vi "KE622x -- Set Lin Log Sweep Params.vi"(0 "Resource In":refnum<visa-resource-name>, 1 "Check For SCPI Errors? (T)":bool=TRUE, 7 "Lin Log Sweep Params In":T1={"Sweep Type"=enum."Linear", "Source Delay (s)"=0.001, "Range Method"=enum."Fixed", "Num Sweeps"=enum."Sweep Count", "Sweep Count"=1, "Start Level (A)"=0.0, "Stop Level (A)"=0.1, "Step Level (A)"=0.01, "Num Steps"=11, "Abort On\nCompliance?"=FALSE} {"Num Steps" min=1 max=65535; "Step Level (A)" min=-0.105 max=0.105 format="%.4p"; "Stop Level (A)" min=-0.105 max=0.105 format="%.4p"; "Start Level (A)" min=-0.105 max=0.105 format="%.4p"; "Sweep Count" min=1 max=9999; "Source Delay (s)" min=0.001 max=1000.0 step=0.001 format="%.3f"}, 11 "error in (no error)":errorcluster, 12 "Read Back Set Values? (T)":bool=TRUE) -> (4 "Resource Out (dupl)":refnum<visa-resource-name>, 8 "Lin Log Sweep Params Out":T1={"Sweep Type"=enum."Linear", "Source Delay (s)"=0.0, "Range Method"=enum."Fixed", "Num Sweeps"=enum."Sweep Count", "Sweep Count"=1, "Start Level (A)"=0.0, "Stop Level (A)"=0.1, "Step Level (A)"=0.01, "Num Steps"=11, "Abort On\nCompliance?"=FALSE} {"Num Steps" min=1 max=65535; "Step Level (A)" min=-0.105 max=0.105 format="%.4p"; "Stop Level (A)" min=-0.105 max=0.105 format="%.4p"; "Start Level (A)" min=-0.105 max=0.105 format="%.4p"; "Sweep Count" min=1 max=9999; "Source Delay (s)" min=0.001 max=1000.0 step=0.001 format="%.3f"}, 15 "error out":errorcluster)   [LabVIEW 2019, in "Keithley 622x.lvlib"]
doc: "Sets the parameters associated with a linear or log current sweep. The user must select the sweep type ('Linear' or 'Log'). Note that 'Step Level (A)' only applies to linear sweeps."
uses:
  Keithley 622x.lvlib
  Typedefs/KE622x -- Lin Log Sweep Params.ctl
  Typedefs/KE622x -- Source Delay.ctl
  Typedefs/KE622x -- Current Level.ctl
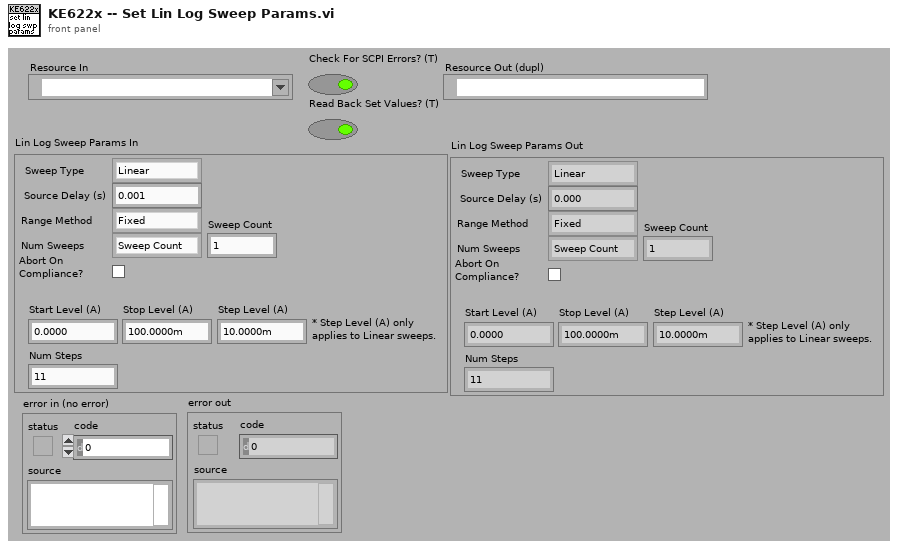
[diagram p1: front panel]
types:
  T1 = typedef "Keithley 622x.lvlib/KE622x -- Lin Log Sweep Params.ctl" = cluster{"Sweep Type":enum16{"Linear", "Log", "List"}, "Source Delay (s)":T2, "Range Method":enum16{"Auto", "Best", "Fixed"}, "Num Sweeps":enum16{"Sweep Count", "Infinite"}, "Sweep Count":u32, "Start Level (A)":T3, "Stop Level (A)":T3, "Step Level (A)":T3, "Num Steps":u32, "Abort On\nCompliance?":bool}
  T2 = typedef "Keithley 622x.lvlib/KE622x -- Source Delay.ctl" = dbl
  T3 = typedef "Keithley 622x.lvlib/KE622x -- Current Level.ctl" = dbl
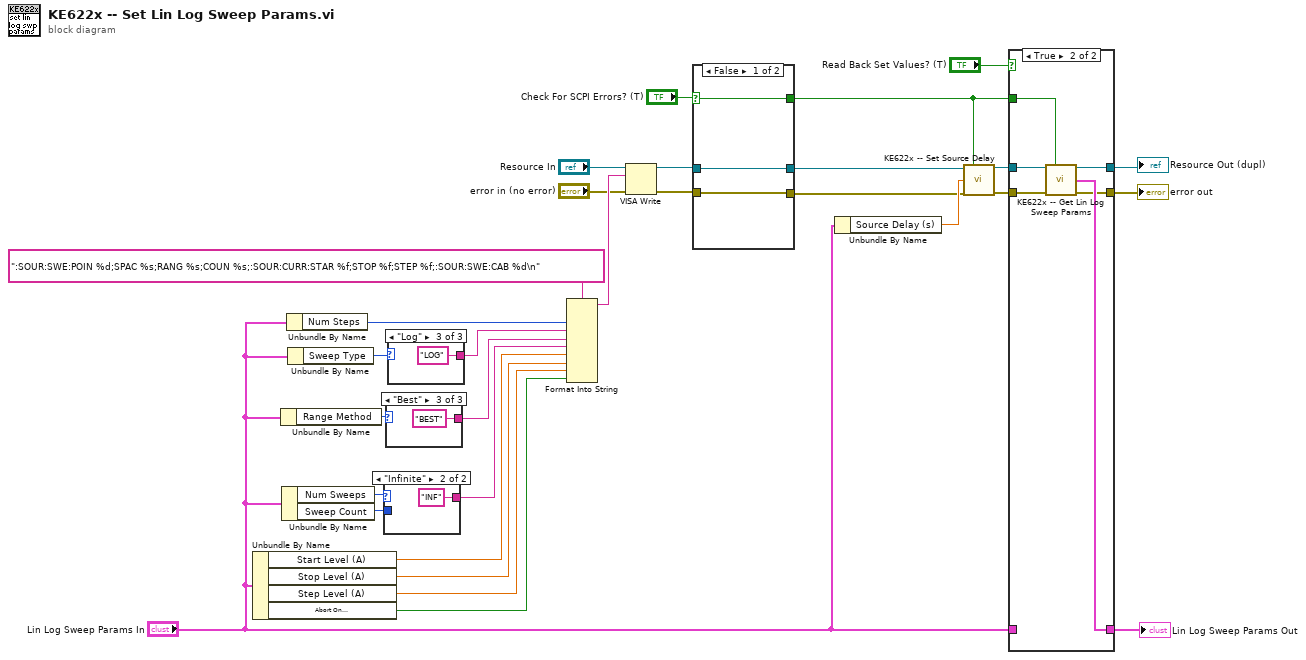
[diagram p0: block diagram]
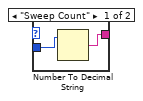
[diagram p3: hidden frame]
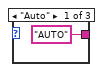
[diagram p4: hidden frame]
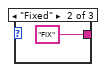
[diagram p5: hidden frame]
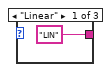
[diagram p6: hidden frame]
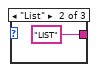
[diagram p7: hidden frame]
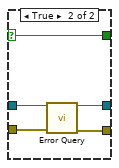
[diagram p8: hidden frame]
diagram:
  n1 = Unbundle By Name("Lin Log Sweep Params In") -> ("Start Level (A)"=w20:T3, "Stop Level (A)"=w19:T3, "Step Level (A)"=w18:T3, "Abort On\nCompliance?"=w1:bool)
  n2 = Unbundle By Name("Lin Log Sweep Params In") -> ("Range Method"=w25:enum16{"Auto", "Best", "Fixed"})
  n3 = Unbundle By Name("Lin Log Sweep Params In") -> ("Num Sweeps"=w23:enum16{"Sweep Count", "Infinite"}, "Sweep Count"=w22:u32)
  n4 = Unbundle By Name("Lin Log Sweep Params In") -> ("Num Steps"=w28:u32)
  n5 = Unbundle By Name("Lin Log Sweep Params In") -> ("Sweep Type"=w27:enum16{"Linear", "Log", "List"})
  n6 = case shown="\"Infinite\"" w23 {
    tunnel: [w31 "INF"] -> w21
    tunnel: w22 -> [w32 _]
    frame "Sweep Count" {
      n7 = Number To Decimal String(number=w32) -> (decimal integer string=w31:string)  [unwired: 1 in]
    }
    frame "Infinite" {
    }
  }
  n8 = case shown="\"Best\"" w25 {
    tunnel: ["AUTO" "FIX" "BEST"] -> w24
    frame "Auto" {
    }
    frame "Fixed" {
    }
    frame "Best" {
    }
  }
  n9 = case shown="\"Log\"" w27 {
    tunnel: ["LIN" "LIST" "LOG"] -> w26
    frame "Linear" {
    }
    frame "List" {
    }
    frame "Log" {
    }
  }
  n10 = Format Into String(format string=":SOUR:SWE:POIN %d;SPAC %s;RANG %s;COUN %s;:SOUR:CURR:STAR %f;STOP %f;STEP %f;:SOUR:SWE:CAB %d\n", w28, w26, w24, w21, w20, w19, w18, w1) -> (resulting string=w29:string)  [unwired: 2 in, 1 out]
  n11 = VISA Write(VISA resource name="Resource In", write buffer=w29, error in (no error)="error in (no error)") -> (VISA resource name out=w14:refnum<visa-resource-name>, error out=w15:errorcluster)  [unwired: 1 out]
  n12 = case shown="False" "Check For SCPI Errors? (T)" {
    selector: "Check For SCPI Errors? (T)" -> [w40 w43]
    tunnel: w14 -> [w42 w47]
    tunnel: w15 -> [w41 w46]
    tunnel: [w41 w45] -> w10
    tunnel: [w42 w44] -> w11
    tunnel: [w40 w43] -> w6
    frame False {
    }
    frame True {
      n13 = call "Error Query.vi"("VISA Resource In"=w47, "error in (no error)"=w46) -> ("VISA Resource Out (dupl)"=w44:refnum<visa-resource-name>, "error out"=w45:errorcluster)  [unwired: 10 in, 2 out]
    }
  }
  n14 = Unbundle By Name("Lin Log Sweep Params In") -> ("Source Delay (s)"=w17:T2)
  n15 = call "KE622x -- Set Source Delay.vi"("Resource In"=w11, "Check For SCPI Errors? (T)"=w6, "Source Delay In (s)"=w17, "error in (no error)"=w10) -> ("Resource Out (dupl)"=w8:refnum<visa-resource-name>, "error out"=w7:errorcluster)  [unwired: 9 in, 1 out]
  n16 = case shown="True" "Read Back Set Values? (T)" {
    tunnel: w8 -> [w49 w56]
    tunnel: w7 -> [w48 w55]
    tunnel: w6 -> [_ w54]
    tunnel: "Lin Log Sweep Params In" -> [w50 _]
    tunnel: [w50 w53] -> w2
    tunnel: [w48 w52] -> w3
    tunnel: [w49 w51] -> w4
    frame False {
    }
    frame True {
      n17 = call "KE622x -- Get Lin Log Sweep Params.vi"("Resource In"=w56, "Check For SCPI Errors? (T)"=w54, "error in (no error)"=w55) -> ("Resource Out (dupl)"=w51:refnum<visa-resource-name>, "Lin Log Sweep Params"=w53:T1, "error out"=w52:errorcluster)  [unwired: 10 in]
    }
  }
  "Resource Out (dupl)" <- w4
  "error out" <- w3
  "Lin Log Sweep Params Out" <- w2
